vi "Close.vi"(8 "error in":errorcluster, 11 "Current Setpoint in":refnum<class "Current Setpoint.lvclass">) -> (0 "error out":errorcluster, 3 "Current Setpoint out":refnum<class "Current Setpoint.lvclass">)   [LabVIEW 2023, in "Current Setpoint.lvclass"]
uses:
  Current Setpoint.lvclass
  Parents/Setpoint/Setpoint.lvclass
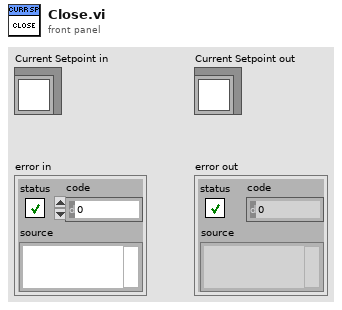
[diagram p1: front panel]
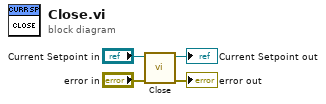
[diagram p0: block diagram]
diagram:
  n1 = call-parent "Close.vi"("error in"="error in", "Setpoint in"="Current Setpoint in") -> ("error out"=→"error out":errorcluster, "Setpoint out"=→"Current Setpoint out":refnum<class "Current Setpoint.lvclass">)  [unwired: 8 in]
